vi "Magazine_Globals.vi"() -> ()   [LabVIEW 2020]
uses:
  Subsystems/Magazine/Magazine_Cluster.ctl
  Subsystems/Magazine/Magazine_Control_States.ctl
  Utility VIs/Basic_Motor_Modes.ctl
panel:
  in  "Magazine_Basic_Motor_Mode":T1
  in  "Magazine_IR":string="Magazine_IR"
  in  "Magazine_Motor_Value":dbl
  in  "Magazine_Execute_Notifier":refnum<notifier>
  in  "Magazine_Set_Notifier":refnum<notifier>
  in  "Magazine_Execute_Ref":string="Magazine_Execute_Ref"
  in  "Magazine_Set_Ref":string="Magazine_Set_Ref"
  in  "Magazine_Motor":string="Magazine_Motor"
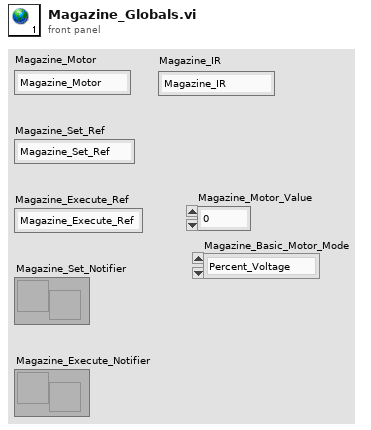
[diagram p1: front panel]
types:
  T1 = typedef "Basic_Motor_Modes.ctl" = enum16{"Percent_Voltage", "Speed_Control", "Position_Control", "Current"}
diagram:
